vi "Basic Waveform Read Example.vi"(8 "error in (no error)":errorcluster) -> (0 "error out":errorcluster)   [LabVIEW 2018]
panel:
  out "Valid Measurements?":bool
  out "Waveform":waveform(dbl)(graph)
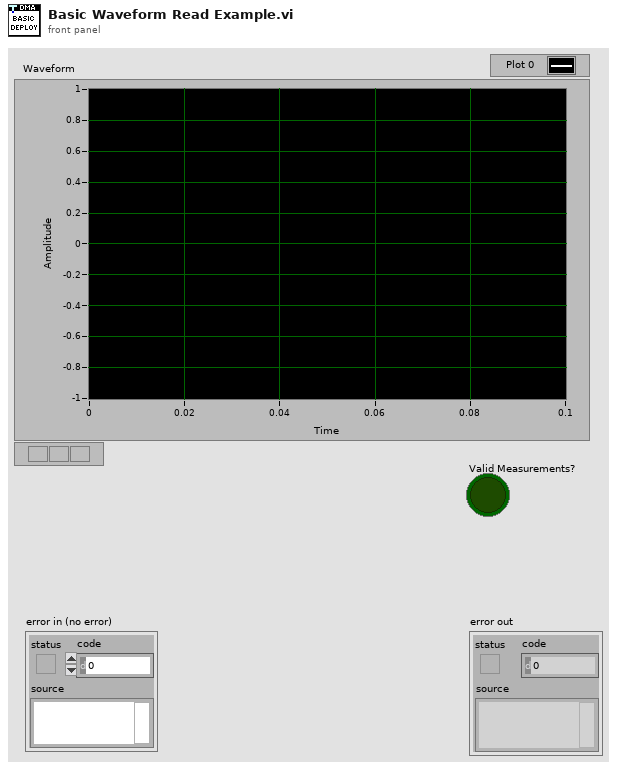
[diagram p1: front panel]
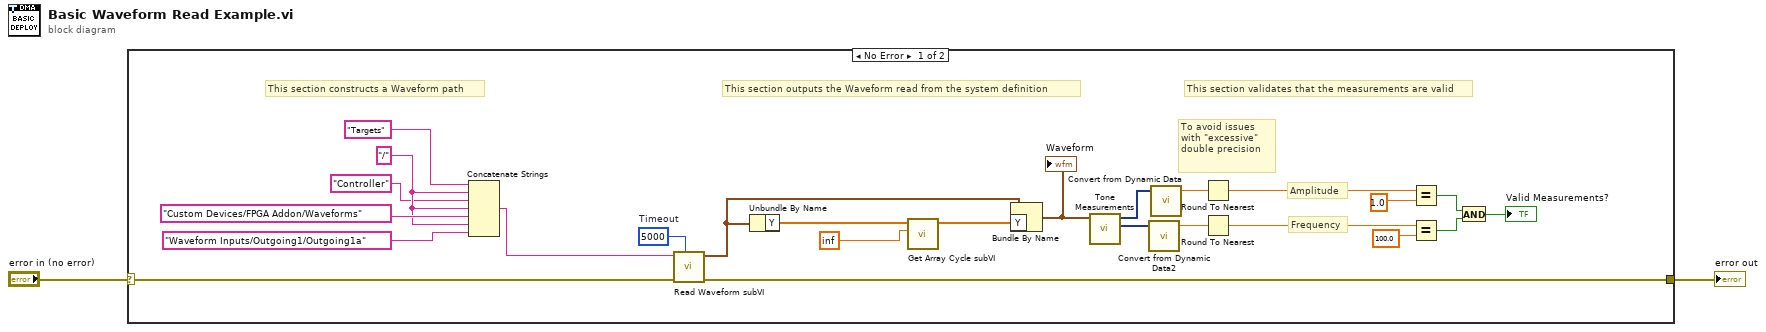
[diagram p0: block diagram]
diagram:
  n1 = case shown="No Error" "error in (no error)" {
    selector: "error in (no error)" -> [w10 w28]
    tunnel: [w9 w28] -> w2
    frame No Error {
      w13 = "/" ("string")
      w7 = 5000  # Timeout
      # "This section validates that the measurements are valid"
      # "This section outputs the Waveform read from the system definition"
      # "This section constructs a Waveform path"
      # "To avoid issues with \"excessive\" double precision"
      # "Frequency"
      # "Amplitude"
      n2 = Concatenate Strings("Targets" ("string"), w13, "Controller" ("Target Name"), w13, "Custom Devices/FPGA Addon/Waveforms" ("string"), w13, "Waveform Inputs/Outgoing1/Outgoing1a" ("Relative Waveform Path")) -> (w8:string)
      n3 = call "Read Waveform subVI.vi"("Timeout"=w7, "error in"=w10, "Waveform Path"=w8) -> ("error out"=w9:errorcluster, "waveform"=w6:waveform(dbl))  [unwired: 7 in]
      n4 = Unbundle By Name(w6) -> ("Y"=w4:dbl[])
      n5 = call "Get Array Cycle subVI.vi"("Marker"=inf, "Array Samples"=w4) -> ("Array"=w5:dbl[])  [unwired: 8 in, 1 out]
      n6 = Bundle By Name(cluster=w6, "Y"=w5) -> (w27:waveform(dbl))
      "Waveform" <- w27
      n7 = call "Tone Measurements"("Signals"=w27) -> ("Frequency"=w26:dynamicdata, "Amplitude"=w25:dynamicdata)  [unwired: 8 in, 1 out]
      n8 = call "Convert from Dynamic Data2"("Dynamic Data Type"=w26) -> ("Scalar"=w23:dbl)  [unwired: 3 in]
      n9 = call "Convert from Dynamic Data"("Dynamic Data Type"=w25) -> ("Scalar"=w24:dbl)  [unwired: 3 in]
      n10 = Round To Nearest(number=w24) -> (nearest integer value=w21:dbl)
      n11 = Round To Nearest(number=w23) -> (nearest integer value=w19:dbl)
      n12 = Equal?(x=w21, y=1.0 ("Scalar")) -> (x = y?=w17:bool)
      n13 = Equal?(x=w19, y=100.0 ("Scalar")) -> (x = y?=w18:bool)
      n14 = And(x=w17, y=w18) -> (x .and. y?=→"Valid Measurements?":bool)
    }
    frame Error {
    }
  }
  "error out" <- w2
